vi "Algae Target Loop.vi"(0 "Camera Name":string="cam0") -> ()   [LabVIEW 2023]
uses:
  State Machine/Ball States.ctl
  State Machine/Ball Main CLuster.ctl
  <vilib>/vision/Image Controls.llb/IMAQ Image.ctl
  Steam Type.ctl
  Camera Set Up/Event Setup Types.ctl
  <vilib>/Utility/config.llb/Read Key (String).vi
  <vilib>/Utility/config.llb/Write Key (String).vi
  <vilib>/Utility/config.llb/NI_LVConfig.lvlib
  <vilib>/vision/NI_Vision_Development_Module.lvlib
panel:
  in  "Main":enum32{"Page 1", "Page 2"}(tab)
  out "Algae Distance":dbl[](array[numeric]) caption="Distance" format="%.1f"
  out "Algae Angle":dbl[](array[numeric]) caption="Angle" format="%.1f"
  out "Image":T1(plugin-control)
  in  "Settings":bool
  in  "Save":bool
  in  "Tools":bool
  out "Ball Fps":dbl format="%#.0f"
  in  "Home":bool
  in  "Ball Diameter (in)":dbl=16.0
  in  "FOV":dbl=68.5
  in  "Algae Color Range":T2={"Hue"={21.620689392089844, 69.62068939208984}, "Sat"={66.41378784179688, 255.0}, "Val"={96.0, 255.0}} caption="Color Range" {"Hue" scale=0.0..255.0 scale format="%#_3g"}
  out "Mask":T1(plugin-control)
  in  "Score Threshold %":dbl=80.0
  # "Edit the camera name to the camera that you are going to use for this target package"
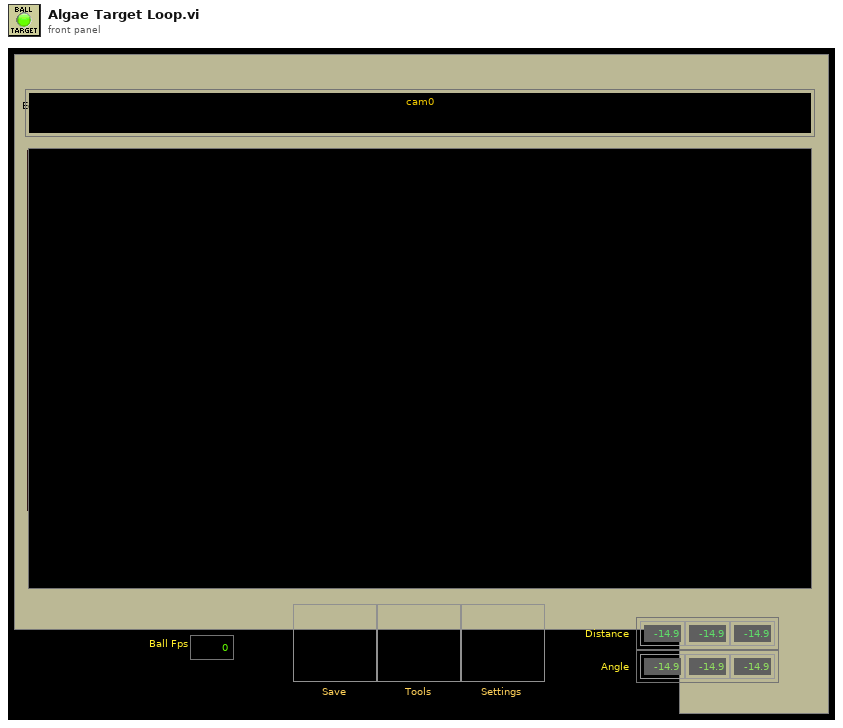
[diagram p1: front panel]
types:
  T1 = typedef "IMAQ Image.ctl" = refnum<image>
  T2 = cluster{"Hue":cluster{dbl, dbl}, "Sat":cluster{dbl, dbl}, "Val":cluster{dbl, dbl}}
  T3 = typedef "Ball Main CLuster.ctl" = cluster{"Ball FIFO":T4[], "Camera Name":string, "Ball path":path, "Control Ref's":refnum<vi>[], "Greyscale Mask Image":T1, "Main Image":T1, "Algae Color Range":cluster{"Hue":cluster{dbl, dbl}, "Sat":cluster{dbl, dbl}, "Val":cluster{dbl, dbl}}, "Timeout":i32}
  T4 = typedef "Ball States.ctl" = enum16{"Message Dispatcher", "INI", "Open", "Save", "Exit"}
  T5 = typedef "Particle Parameters" = i32
  T6 = typedef "Steam Type.ctl" = enum8{"Unknown", "Apriltag", "Algae", "Coral"}
  T7 = typedef "Event Setup Types.ctl" = enum16{"Default", "Camera Loop Started", "Save Data", "Open Front Panel", "Exit"}
  T8 = typedef "Target Fields.ctl" = cluster{"diameter points":cluster{"first point":cluster{"x":dbl, "y":dbl}, "projected point":cluster{"x":dbl, "y":dbl}}, "normalized center":cluster{"x":dbl, "y":dbl}, "Overall Score":dbl, "Area Score":dbl, "Moment Score":dbl, "Aspect Score":dbl, "Distance (ft)":dbl, "Upper Goal":bool}
  T9 = cluster{cluster{"Lower":dbl, "Upper":dbl}, cluster{"Lower":dbl, "Upper":dbl}, cluster{"Lower":dbl, "Upper":dbl}}
  T10 = typedef "Image Type" = u32
  T11 = typedef "NI_LVConfig.lvlib/Config Data RefNum.ctl" = refnum<k1>
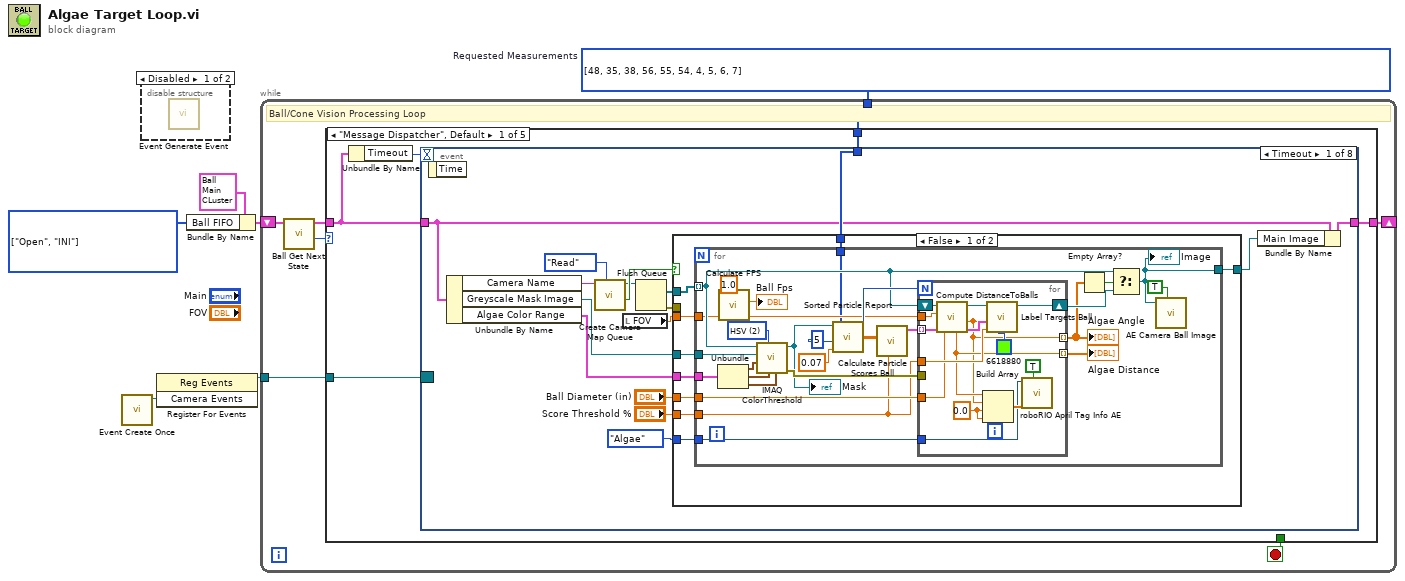
[diagram p0: block diagram]
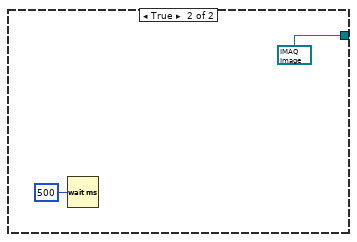
[diagram p3: hidden frame]
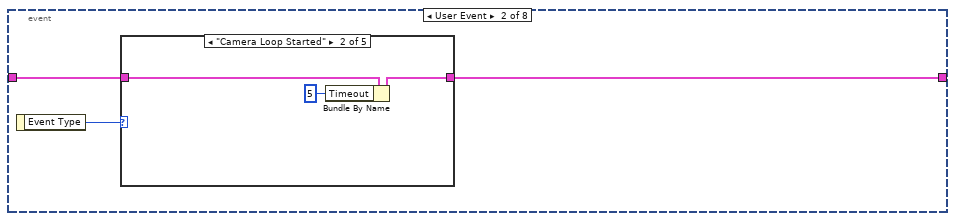
[diagram p4: hidden frame]
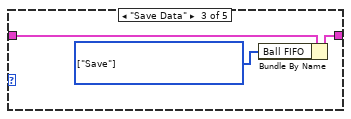
[diagram p6: hidden frame]
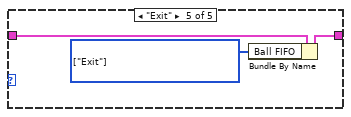
[diagram p8: hidden frame]
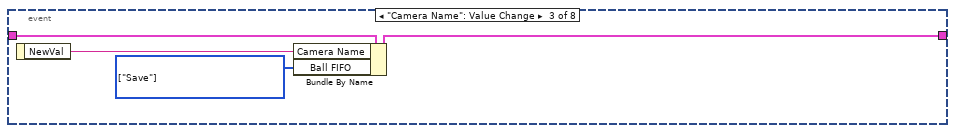
[diagram p9: hidden frame]
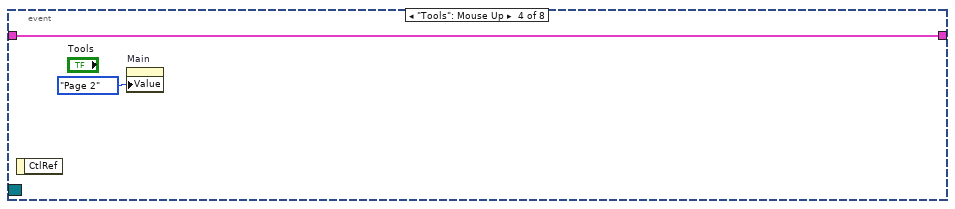
[diagram p10: hidden frame]
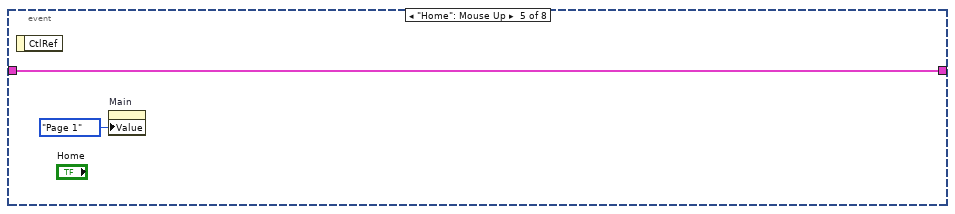
[diagram p11: hidden frame]
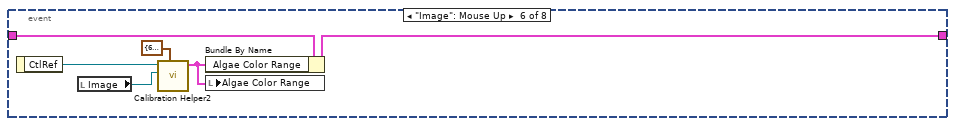
[diagram p12: hidden frame]
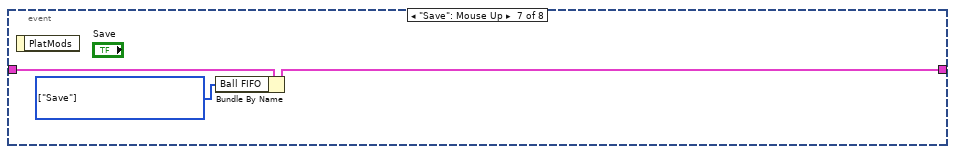
[diagram p13: hidden frame]
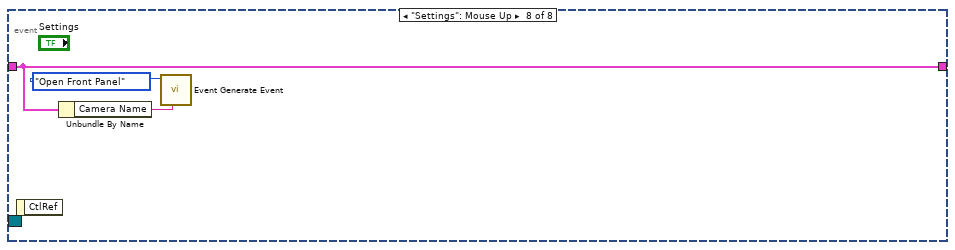
[diagram p14: hidden frame]
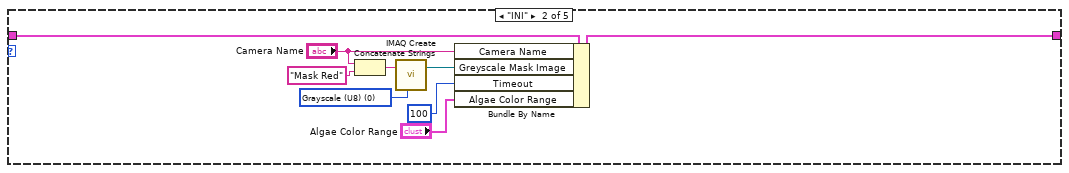
[diagram p15: hidden frame]
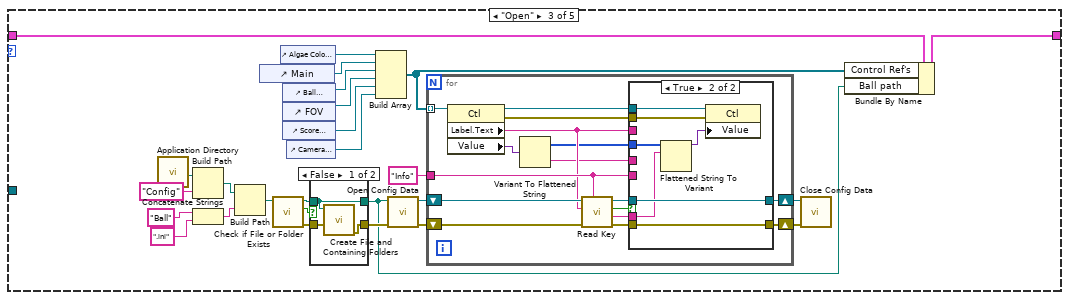
[diagram p16: hidden frame]
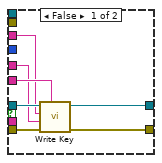
[diagram p18: hidden frame]
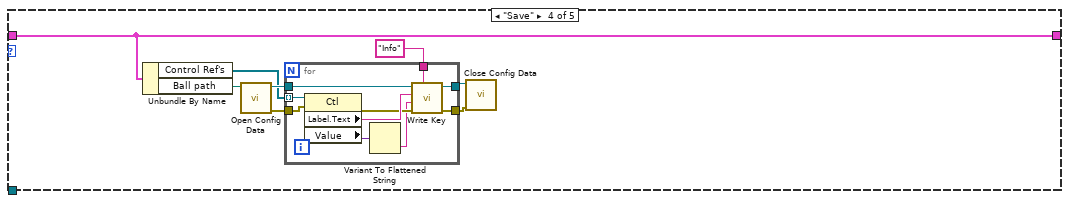
[diagram p19: hidden frame]
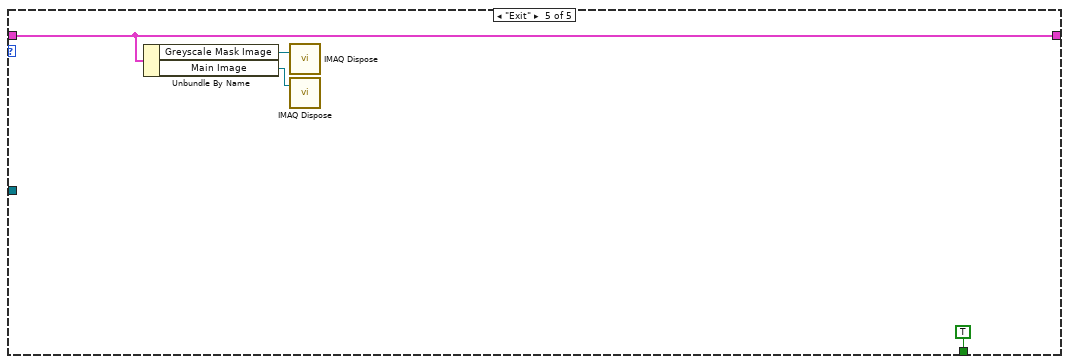
[diagram p20: hidden frame]
diagram:
  w2 = T4[] [enum."Open", enum."INI"] items=["Message Dispatcher", "INI", "Open", "Save", "Exit"] ("Ball FIFO")
  w4 = T5[] [48, 35, 38, 56, 55, 54, 4, 5, 6, 7] items=["Center of Mass X", "Center of Mass Y", "First Pixel X", "First Pixel Y", "Bounding Rect Left", "Bounding Rect Top", "Bounding Rect Right", "Bounding Rect Bottom", "Max Feret Diameter Start X", "Max Feret Diameter Start Y", "Max Feret Diameter End X", "Max Feret Diameter End Y", "Max Horiz. Segment Length Left", "Max Horiz. Segment Length Right", "Max Horiz. Segment Length Row", "-", "Bounding Rect Width", "Bounding Rect Height", "Bounding Rect Diagonal", "Perimeter", "Convex Hull Perimeter", "Holes' Perimeter", "Max Feret Diameter", "Equivalent Ellipse Major Axis", "Equivalent Ellipse Minor Axis", "Equivalent Ellipse Minor Axis (Feret)", "Equivalent Rect Long Side", "Equivalent Rect Short Side", "Equivalent Rect Diagonal", "Equivalent Rect Short Side (Feret)", "Average Horiz. Segment Length", "Average Vert. Segment Length", "Hydraulic Radius", "Waddel Disk Diameter", "-", "Area", "Holes' Area", "Particle & Holes' Area", "Convex Hull Area", "Image Area", "-", "Number of Holes", "Number of Horiz. Segments", "Number of Vert. Segments", "-", "Orientation", "Max Feret Diameter Orientation", "-", "% Area/Image Area", "% Area/(Particle & Holes' Area)", "Ratio of Equivalent Ellipse Axes", "Ratio of Equivalent Rect Sides", "-", "Elongation Factor", "Compactness Factor", "Heywood Circularity Factor", "Type Factor", "-", "Sum X", "Sum Y", "Sum XX", "Sum XY", "Sum YY", "Sum XXX", "Sum XXY", "Sum XYY", "Sum YYY", "-", "Moment of Inertia XX", "Moment of Inertia XY", "Moment of Inertia YY", "Moment of Inertia XXX", "Moment of Inertia XXY", "Moment of Inertia XYY", "Moment of Inertia YYY", "Norm. Moment of Inertia XX", "Norm. Moment of Inertia XY", "Norm. Moment of Inertia YY", "Norm. Moment of Inertia XXX", "Norm. Moment of Inertia XXY", "Norm. Moment of Inertia XYY", "Norm. Moment of Inertia YYY", "Hu Moment 1", "Hu Moment 2", "Hu Moment 3", "Hu Moment 4", "Hu Moment 5", "Hu Moment 6", "Hu Moment 7"]  # Requested Measurements
  n1 = call "Event Create Once.vi"() -> ("Camera Events"=w6:refnum<user-event>)  [unwired: 10 in, 1 out]
  n2 = disable-structure shown="Disabled" {
    frame Disabled {
      n3 = call "Event Generate Event.vi"() -> ()  [unwired: 12 in]
    }
    frame Enabled {
    }
  }
  n4 = register-events(w6) -> (reference out=w5:refnum<event-registration>)  [unwired: 2 in, 1 out]
  n5 = Bundle By Name(cluster=T3 {"Ball FIFO"=[], "Camera Name"="", "Ball path"=path "", "Control Ref's"=[], "Greyscale Mask Image"=refnum, "Main Image"=refnum, "Algae Color Range"={"Hue"={21.620689392089844, 69.62068939208984}, "Sat"={66.41378784179688, 255.0}, "Val"={96.0, 255.0}}, "Timeout"=5} ("Ball Main Cluster in"), "Ball FIFO"=w2) -> (w3:T3)
  n6 = while {
    tunnel: w4 -> [w13]
    tunnel: w5 -> [w12]
    shift-right: [w7] -> _
    shift-left: w3 -> [w10]
    stop <- w11 stop-if-true
    # "Ball/Cone Vision Processing Loop"
    n7 = call "Ball Get Next State.vi"("Ball Main Cluster in"=w10) -> ("Next State"=w9:T4, "Ball Main Cluster out"=w8:T3)  [unwired: 9 in]
    n8 = case shown="\"Message Dispatcher\", Default" w9 {
      tunnel: w13 -> [w18 _ _ _ _]
      tunnel: w12 -> [w17 _ _ _ _]
      tunnel: [_ _ _ _ TRUE] -> w11
      tunnel: w8 -> [w15 w127 w140 w194 w211]
      tunnel: [w16 w126 w138 w194 w211] -> w7
      frame "Message Dispatcher", Default {
        n9 = Unbundle By Name(w15) -> ("Timeout"=w14:i32)
        n10 = event shown="[0] Timeout" {
          selector: w17 -> [_ _ _ _ _ _ _ _]
          dyn-events: _ -> [_ _ _ _ _ _ _ _]
          timeout: w14 -> [_ _ _ _ _ _ _ _]
          tunnel: w18 -> [w34 _ _ _ _ _ _ _]
          tunnel: w15 -> [w23 w90 w105 w106 w108 w112 w118 w120]
          tunnel: [w22 w88 w104 w106 w108 w111 w117 w120] -> w16
          event Timeout {
            n11 = event-data() -> ()  [unwired: 1 in, 1 out]
            n12 = Unbundle By Name(w23) -> ("Camera Name"=w25:string, "Greyscale Mask Image"=w24:T1, "Algae Color Range"=w20:T2)
            n13 = call "Create Camera Map Queue.vi"("Action"=enum16{"Read", "Write"}."Read", "Camera"=w25) -> ("key not found?"=w32:bool, "value"=w28:refnum<queue>)  [unwired: 8 in]
            n14 = local read "FOV"() -> (w31:dbl)
            n15 = Flush Queue(queue=w28) -> (remaining elements=w27:T1[], error out=w26:errorcluster)  [unwired: 1 in, 1 out]
            n16 = case shown="False" w32 {
              tunnel: w34 -> [w43 _]
              tunnel: [w42 T1 refnum ("Image")] -> w21
              tunnel: w24 -> [w41 _]
              tunnel: w31 -> [w40 _]
              tunnel: w20 -> [w39 _]
              tunnel: "Ball Diameter (in)" -> [w38 _]
              tunnel: "Score Threshold %" -> [w37 _]
              tunnel: w27 -> [w36 _]
              tunnel: w26 -> [_ _]
              tunnel: Steam_Type."Algae" ("Stream Type") -> [w35 _]
              frame False {
                n17 = for {
                  tunnel: w41 -> [w65]
                  tunnel: w43 -> [w54]
                  tunnel: w36 -> [w56] mode=indexing
                  tunnel: [w53] -> w42
                  tunnel: w40 -> [w55]
                  tunnel: w39 -> [w60]
                  tunnel: w38 -> [w50]
                  tunnel: w37 -> [w48]
                  tunnel: w35 -> [w44]
                  w66 = u16 2 items=["RGB", "HSL", "HSV", "HSI"] ("Color Mode")
                  n18 = Unbundle(w60) -> ("Hue"=w59:cluster{dbl, dbl}, "Sat"=w58:cluster{dbl, dbl}, "Val"=w57:cluster{dbl, dbl})
                  n19 = call "Calculate FPS.vi"("Frames Processed"=1.0) -> ("Fps"=→"Ball Fps":dbl)  [unwired: 10 in]
                  n20 = call "IMAQ ColorThreshold"("Blue or Luma or Val or Inten Range"=w57, "Green or Sat Range"=w58, "Color Mode"=w66, "Red or Hue Range"=w59, "Image Dst"=w65, "Image Src"=w56) -> ("error out"=w64:errorcluster, "Image Dst Out"=w49:T1)  [unwired: 4 in]
                  "Mask" <- w49
                  n21 = call "Sorted Particle Report.vi"("Min Area Size %"=0.07 ("Size Limit %"), "Particle Count Limit"=5 ("Particle Count LImit"), "Pixel Measurements"=w54, "Image in"=w49) -> ("Sorted Data"=w69:dbl[][], "Particles"=w63:i32)  [unwired: 1 out]
                  n22 = call "Calculate Particle Scores Ball.vi"("Limit"=w48, "Sorted Data"=w69) -> ("Scores"=w68:T8[])  [unwired: 9 in]
                  n23 = for {
                    N: w63 -> [_]
                    tunnel: w68 -> [w83] mode=indexing
                    shift-right: [w85] -> w62
                    shift-left: w56 -> [w81]
                    tunnel: w48 -> [w84]
                    tunnel: [w74] -> w52 mode=indexing
                    tunnel: w64 -> [_]
                    tunnel: w55 -> [w79]
                    tunnel: [w75] -> w51 mode=indexing
                    tunnel: w50 -> [w77]
                    tunnel: w44 -> [w71]
                    w72 = 0.0 ("element")
                    n24 = call "Compute DistanceToBalls.vi"("Target Width (in)"=w77, "results"=w83, "FOV"=w79, "Image Src"=w81) -> ("results out"=w80:T8, "Off Angle"=w74:dbl, "Image Dst Out"=w82:T1, "Distance"=w75:dbl)  [unwired: 3 in, 1 out]
                    n25 = Build Array(w75, w74, w72, w72) -> (w73:dbl[])
                    n26 = call "Label Targets Ball.vi"("Color"=u32 6618880, "Score Threshold"=w84, "results"=w80, "Angle"=w74, "Image in"=w82) -> ("Image out"=w85:T1)  [unwired: 6 in]
                    n27 = call "roboRIO April Tag Info AE.vi"("Update"=TRUE, "Info in"=w73, "Stream Type"=w71) -> ()  [unwired: 8 in, 1 out]
                  }
                  "Algae Angle" <- w52
                  "Algae Distance" <- w51
                  n28 = Empty Array?(array=w52) -> (empty?=w61:bool)
                  n29 = Select(t=w56, s=w61, f=w62) -> (s? t:f=w53:T1)
                  "Image" <- w53
                  n30 = call "AE Camera Ball Image.vi"("Update"=TRUE, "Ball Image in"=w53) -> ()  [unwired: 9 in, 1 out]
                }
              }
              frame True {
                n31 = Wait (ms)(milliseconds to wait=u32 500) -> ()  [unwired: 1 out]
              }
            }
            n32 = Bundle By Name(cluster=w23, "Main Image"=w21) -> (w22:T3)
          }
          event User Event {
            n33 = event-data() -> ("Event Type"=w89:T7)  [unwired: 1 in]
            n34 = case shown="\"Camera Loop Started\"" w89 {
              tunnel: w90 -> [w91 w94 w97 w98 w101]
              tunnel: [w91 w93 w96 w98 w100] -> w88
              frame "Default", Default {
              }
              frame "Camera Loop Started" {
                n35 = Bundle By Name(cluster=w94, "Timeout"=5) -> (w93:T3)
              }
              frame "Save Data" {
                w95 = T4[] [enum."Save"] items=["Message Dispatcher", "INI", "Open", "Save", "Exit"] ("Ball FIFO")
                n36 = Bundle By Name(cluster=w97, "Ball FIFO"=w95) -> (w96:T3)
              }
              frame "Open Front Panel" {
              }
              frame "Exit" {
                w99 = T4[] [enum."Exit"] items=["Message Dispatcher", "INI", "Open", "Save", "Exit"] ("Ball FIFO")
                n37 = Bundle By Name(cluster=w101, "Ball FIFO"=w99) -> (w100:T3)
              }
            }
          }
          event "Camera Name": Value Change {
            w102 = T4[] [enum."Save"] items=["Message Dispatcher", "INI", "Open", "Save", "Exit"] ("Ball FIFO")
            n38 = event-data() -> ("NewVal"=w103:string)  [unwired: 1 in]
            n39 = Bundle By Name(cluster=w105, "Camera Name"=w103, "Ball FIFO"=w102) -> (w104:T3)
          }
          event "Tools": Mouse Up {
            n40 = event-data() -> ()  [unwired: 1 in, 1 out]
            n41 = property on="Main" class="TabCtl (strict)"("Value"=enum32{"Page 1", "Page 2"}."Page 2" ("Main")) -> ()  [unwired: 2 in, 2 out]
          }
          event "Home": Mouse Up {
            n42 = event-data() -> ()  [unwired: 1 in, 1 out]
            n43 = property on="Main" class="TabCtl (strict)"("Value"=enum32{"Page 1", "Page 2"}."Page 1" ("Main")) -> ()  [unwired: 2 in, 2 out]
          }
          event "Image": Mouse Up {
            n44 = event-data() -> ("CtlRef"=w114:refnum<vi>)  [unwired: 1 in]
            n45 = local read "Image"() -> (w113:T1)
            n46 = call "Calibration Helper2.vi"("Std Devs"=cluster{"H":dbl, "S":dbl, "V":dbl} {"H"=6.0, "S"=6.0, "V"=6.0} ("Std Devs Ball"), "Image"=w113, "Image Ctl Refnum"=w114) -> ("output color"=w110:T9)  [unwired: 7 in, 1 out]
            n47 = Bundle By Name(cluster=w112, "Algae Color Range"=w110) -> (w111:T3)
            n48 = local write "Algae Color Range"(w110) -> ()
          }
          event "Save": Mouse Up {
            w116 = T4[] [enum."Save"] items=["Message Dispatcher", "INI", "Open", "Save", "Exit"] ("Ball FIFO")
            n49 = event-data() -> ()  [unwired: 1 in, 1 out]
            n50 = Bundle By Name(cluster=w118, "Ball FIFO"=w116) -> (w117:T3)
          }
          event "Settings": Mouse Up {
            n51 = event-data() -> ()  [unwired: 1 in, 1 out]
            n52 = Unbundle By Name(w120) -> ("Camera Name"=w119:string)
            n53 = call "Event Generate Event.vi"("Camera Name"=w119, "Event Type"=Event_Setup_Types."Open Front Panel") -> ()  [unwired: 10 in]
          }
        }
      }
      frame "INI" {
        w128 = T10 0 items=["Grayscale (U8)", "Grayscale (I16)", "Grayscale (SGL)", "Complex (CSG)", "RGB (U32)", "HSL (U32)", "RGB (U64)", "Grayscale (U16)"] ("Image Type")
        n54 = Concatenate Strings("Camera Name", "Mask Red" ("string")) -> (w130:string)
        n55 = call "IMAQ Create"("Image Name"=w130, "Image Type"=w128) -> ("New Image"=w124:T1)  [unwired: 2 in, 2 out]
        n56 = Bundle By Name(cluster=w127, "Camera Name"="Camera Name", "Greyscale Mask Image"=w124, "Timeout"=100, "Algae Color Range"="Algae Color Range") -> (w126:T3)
      }
      frame "Open" {
        n57 = call <vilib>:"Application Directory.vi"() -> ("Application Directory"=w143:path)
        n58 = Build Path(base path=w143, name or relative path="Config") -> (appended path=w141:path)
        n59 = Concatenate Strings("Ball" ("string"), ".ini" ("name or relative path")) -> (w156:string)
        n60 = Build Path(base path=w141, name or relative path=w156) -> (appended path=w136:path)
        n61 = control-ref of="Main"() -> (w149:refnum<vi>)
        n62 = call <vilib>:"Check if File or Folder Exists.vi"("path"=w136) -> ("error out"=w132:errorcluster, "file or folder exists?"=w134:bool, "dup path"=w135:path)  [unwired: 8 in]
        n63 = control-ref of="Algae Color Range"() -> (w150:refnum<vi>)
        n64 = control-ref of="Ball Diameter (in)"() -> (w148:refnum<vi>)
        n65 = control-ref of="FOV"() -> (w147:refnum<vi>)
        n66 = control-ref of="Score Threshold %"() -> (w146:refnum<vi>)
        n67 = control-ref of="Camera Name"() -> (w131:refnum<vi>)
        n68 = case shown="False" w134 {
          tunnel: [w159 w160] -> w144
          tunnel: w135 -> [w158 w161]
          tunnel: [w158 w161] -> w133
          tunnel: w132 -> [w157 w160]
          frame False {
            n69 = call <vilib>:"Create File and Containing Folders.vi"("error in (no error)"=w157, "file path"=w158) -> ("error out"=w159:errorcluster)  [unwired: 8 in, 1 out]
          }
          frame True {
          }
        }
        n70 = Build Array(w150, w149, w148, w147, w146, w131) -> (w137:refnum<vi>[])
        n71 = call <vilib>:"Open Config Data.vi"("error in (no error)"=w144, "configuration file path"=w133) -> ("error out"=w151:errorcluster, "refnum"=w155:T11)  [unwired: 7 in, 1 out]
        n72 = for {
          tunnel: "Info" ("Camera Name") -> [w174]
          tunnel: w137 -> [w164] mode=indexing
          shift-right: [w176] -> w154
          shift-left: w155 -> [w177]
          shift-right: [w175] -> w153
          shift-left: w151 -> [w173]
          n73 = property class="Ctl"(reference=w164) -> (reference out=w170:refnum<vi>, error out=w169:errorcluster, "Label.Text"=w167:string, "Value"=w163:variant)  [unwired: 1 in]
          n74 = Variant To Flattened String(Variant=w163) -> (data string=w165:string, 1:w162:i16[])
          n75 = call-poly <vilib>:"Read Key.vi"("section"=w174, "error in (no error)"=w173, "key"=w167, "refnum"=w177) -> ("error out"=w166:errorcluster, "value"=w171:string, "found?"=w172:bool, "refnum out"=w168:T11)  [unwired: 4 in]
          n76 = case shown="True" w172 {
            tunnel: w171 -> [_ w186]
            tunnel: w170 -> [_ w191]
            tunnel: w169 -> [_ w190]
            tunnel: w168 -> [w184 w189]
            tunnel: w174 -> [w183 _]
            tunnel: w167 -> [w182 _]
            tunnel: [w181 w189] -> w176
            tunnel: w166 -> [w180 w188]
            tunnel: [w179 w188] -> w175
            tunnel: w165 -> [w178 _]
            tunnel: w162 -> [_ w185]
            frame False {
              n77 = call-poly <vilib>:"Write Key.vi"("section"=w183, "error in (no error)"=w180, "value"=w178, "key"=w182, "refnum"=w184) -> ("error out"=w179:errorcluster, "refnum out"=w181:T11)  [unwired: 4 in, 1 out]
            }
            frame True {
              n78 = Flattened String To Variant(6:w186, 7:w185) -> (3:w187:variant)  [unwired: 1 in, 1 out]
              n79 = property class="Ctl"(reference=w191, error in=w190, "Value"=w187) -> ()  [unwired: 2 out]
            }
          }
        }
        n80 = call <vilib>:"Close Config Data.vi"("error in (no error)"=w153, "refnum"=w154) -> ()  [unwired: 8 in, 2 out]
        n81 = Bundle By Name(cluster=w140, "Control Ref's"=w137, "Ball path"=w133) -> (w138:T3)
      }
      frame "Save" {
        n82 = Unbundle By Name(w194) -> ("Control Ref's"=w192:refnum<vi>[], "Ball path"=w193:path)
        n83 = call <vilib>:"Open Config Data.vi"("configuration file path"=w193) -> ("error out"=w198:errorcluster, "refnum"=w199:T11)  [unwired: 8 in, 1 out]
        n84 = for {
          tunnel: w192 -> [w209] mode=indexing
          tunnel: w199 -> [w208]
          tunnel: w198 -> [w207]
          tunnel: "Info" ("Camera Name") -> [w203]
          tunnel: [w201] -> w197
          tunnel: [w200] -> w196
          n85 = property class="Ctl"(reference=w209, error in=w207) -> (error out=w204:errorcluster, "Label.Text"=w206:string, "Value"=w205:variant)  [unwired: 1 out]
          n86 = Variant To Flattened String(Variant=w205) -> (data string=w202:string)  [unwired: 1 out]
          n87 = call-poly <vilib>:"Write Key.vi"("section"=w203, "error in (no error)"=w204, "value"=w202, "key"=w206, "refnum"=w208) -> ("error out"=w201:errorcluster, "refnum out"=w200:T11)  [unwired: 4 in, 1 out]
        }
        n88 = call <vilib>:"Close Config Data.vi"("error in (no error)"=w197, "refnum"=w196) -> ()  [unwired: 8 in, 2 out]
      }
      frame "Exit" {
        n89 = Unbundle By Name(w211) -> ("Greyscale Mask Image"=w213:T1, "Main Image"=w212:T1)
        n90 = call "IMAQ Dispose"("Image"=w213) -> ()  [unwired: 5 in, 1 out]
        n91 = call "IMAQ Dispose"("Image"=w212) -> ()  [unwired: 5 in, 1 out]
      }
    }
  }
